vi "Write_Instr.vi"(8 "error in (no error)":errorcluster caption="entrée d'erreur (pas d'erreur)", 11 "Class Multimeter (Default) en entrée":refnum<class "Class Instrument Printer.lvclass">) -> (0 "error out":errorcluster caption="sortie d'erreur", 3 "Class Multimeter (Default) en sortie":refnum<class "Class Instrument Printer.lvclass">)   [LabVIEW 2020, in "Library Instrument & Equipement.lvlib" / "Library Instruments.lvlib" / "Class Instrument Printer.lvclass"]
uses:
  Class Instrument Printer.lvclass
  Class Instrument Printer.lvclass/Class Instrument Printer.ctl
  Instrument (Default)/Class Instrument (Default).lvclass
  Printer/Printer (Default)/Class Printer (Default).lvclass
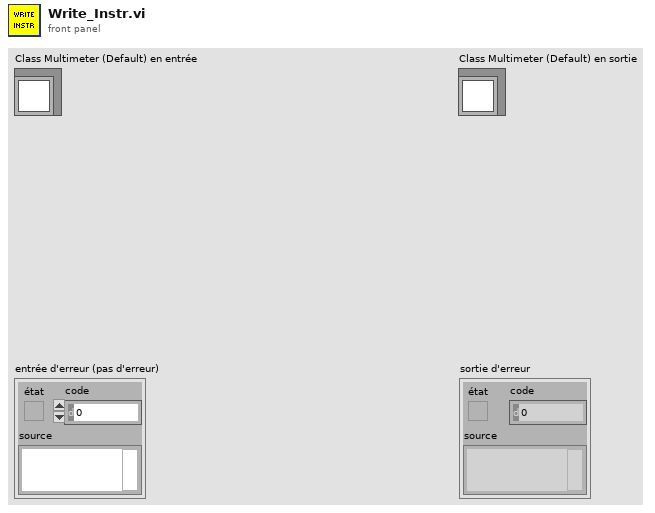
[diagram p1: front panel]
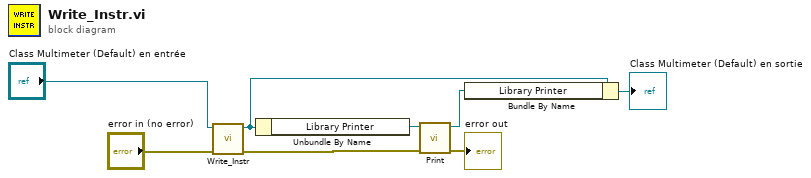
[diagram p0: block diagram]
diagram:
  n1 = call-parent "Write_Instr.vi"("error in (no error)"="error in (no error)", "Class Multimeter (Default) en entrée"="Class Multimeter (Default) en entrée") -> ("error out"=w1:errorcluster, "Class Multimeter (Default) en sortie"=w3:refnum<class "Class Instrument Printer.lvclass">)  [unwired: 8 in]
  n2 = Unbundle By Name(w3) -> ("Library Printer"=w2:refnum<class "Class Printer (Default).lvclass">)
  n3 = call-dynamic "Print.vi"("error in (no error)"=w1, "Class Printer (Default) en entrée"=w2) -> ("error out"=→"error out":errorcluster, "Class Printer (Default) en sortie"=w6:refnum<class "Class Printer (Default).lvclass">)  [unwired: 8 in]
  n4 = Bundle By Name(cluster=w3, "Library Printer"=w6) -> (→"Class Multimeter (Default) en sortie":refnum<class "Class Instrument Printer.lvclass">)
